vi "uDAQtester.vi"() -> ()   [LabVIEW 2017]
uses:
  <vilib>/Math Plots/3D Math Plots/3D Surface/3D Surface XCtrl/3D Surface.xctl
  <vilib>/Math Plots/3D Math Plots/3D Surface/3D Surface Datatype/Public/Plot Helper (Matrix).vi
  <vilib>/Math Plots/3D Math Plots/3D Surface/3D Surface Datatype/3D Surface Datatype.lvclass
panel:
  out "MWTP":dbl
  out "Channel 64":dbl
  out "3D Surface":refnum<class "3D Plot Datatype.lvclass">[](xcontrol)
  in  "Frequency (Hz)":dbl format="%#_13g"
  in  "Samples":i32
  in  "Stop Button":bool
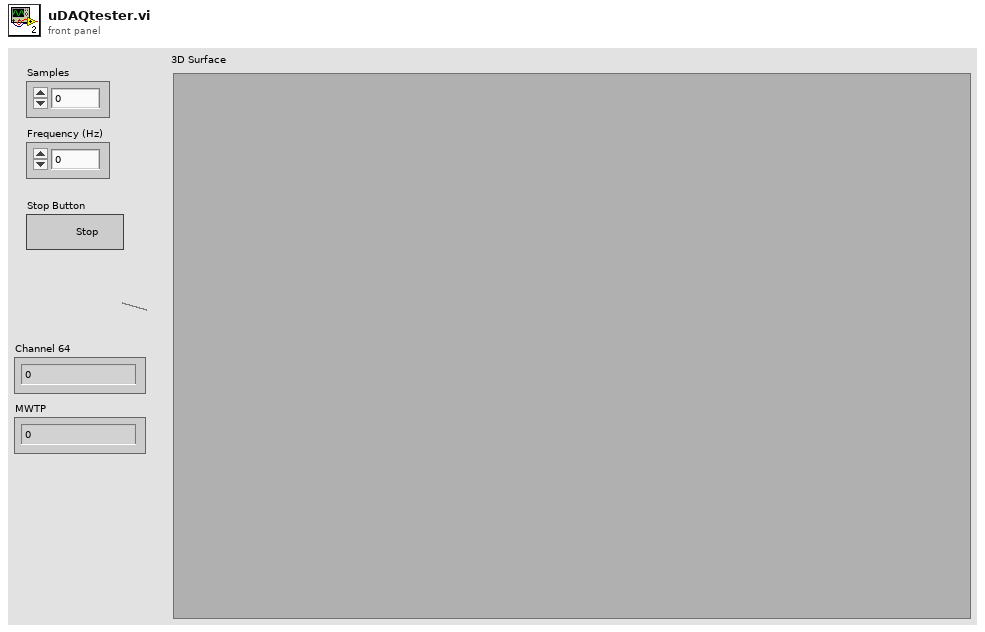
[diagram p1: front panel]
types:
  T1 = typedef "Real Matrix NI_Silver.ctl" = dbl[][]
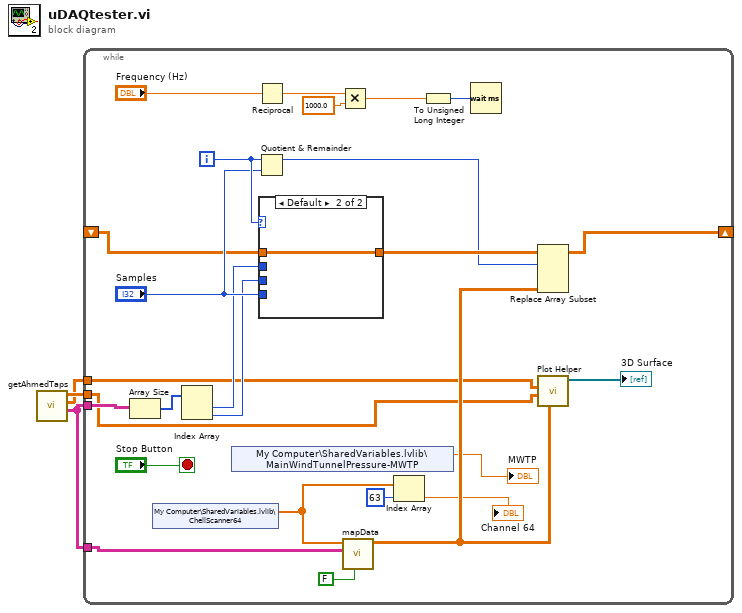
[diagram p0: block diagram]
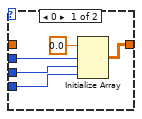
[diagram p2: hidden frame]
diagram:
  n1 = call "getAhmedTaps.vi"() -> ("MAP"=w3:string[][], "Y"=w1:dbl[][], "X"=w2:dbl[][])  [unwired: 7 in]
  n2 = while {
    shift-right: [w13] -> _
    shift-left: _ -> [w20]
    tunnel: w3 -> [w18]
    tunnel: w3 -> [w17]
    tunnel: w2 -> [w8]
    tunnel: w1 -> [w9]
    i -> [w23]
    stop <- "Stop Button" stop-if-true
    n3 = Array Size(array=w17) -> (size(s)=w22:i32[])
    n4 = shared-variable "My Computer\\SharedVariables.lvlib\\ChellScanner64"() -> (w7:dbl[])  [unwired: 1 in, 1 out]
    n5 = Index Array(array=w22) -> (element #1=w15:i32, element #2=w14:i32)  [unwired: 2 in]
    n6 = shared-variable "My Computer\\SharedVariables.lvlib\\MainWindTunnelPressure-MWTP"() -> (→"MWTP":dbl)  [unwired: 1 in, 1 out]
    n7 = Reciprocal(x="Frequency (Hz)") -> (1/x=w28:dbl)
    n8 = Quotient & Remainder(x=w23, y="Samples") -> (x-y*floor(x/y)=w16:i32)  [unwired: 1 out]
    n9 = case shown="Default" w23 {
      tunnel: [w30 w35] -> w19
      tunnel: w15 -> [w34 _]
      tunnel: w14 -> [w33 _]
      tunnel: "Samples" -> [w32 _]
      tunnel: w20 -> [_ w35]
      frame 0 {
        n10 = Initialize Array(0.0 ("element"), w34, w33, w32) -> (w30:dbl[][][])
      }
      frame Default {
      }
    }
    n11 = Multiply(x=w28, y=1000.0) -> (x*y=w26:dbl)
    n12 = call "mapData.vi"("Zero Index"=FALSE, "MAP"=w18, "1D Data"=w7) -> ("Real Matrix"=w10:T1)  [unwired: 8 in]
    n13 = Index Array(array=w7, index=63) -> (element=→"Channel 64":dbl)
    n14 = To Unsigned Long Integer(number=w26) -> (unsigned 32bit integer=w25:u32)
    n15 = Wait (ms)(milliseconds to wait=w25) -> ()  [unwired: 1 out]
    n16 = Replace Array Subset(array=w19, new element=w10, index (dim 0)=w16) -> (w13:dbl[][][])  [unwired: 2 in]
    n17 = call-poly <vilib>:"Plot Helper.vi"("z matrix"=w10, "y matrix"=w8, "x matrix"=w9) -> ("3D Plot lvclass Array out"=→"3D Surface":refnum<class "3D Plot Datatype.lvclass">[])  [unwired: 3 in, 5 out]
  }
